vi "test_Basic Deployment.vi"(8 "error in (no error)":errorcluster, 11 "TestCase in":refnum<class "Telemetry System Tests.lvclass">) -> (0 "error out":errorcluster, 3 "TestCase out":refnum<class "Telemetry System Tests.lvclass">)   [LabVIEW 2019, in "Telemetry System Tests.lvclass"]
uses:
  Telemetry System Tests.lvclass
  C:/Users/nitest/Desktop/NI VS Custom Device Testing Tools/VeriStandTestCase/VeriStandTestCase.lvclass
  NI VS Custom Device Testing Tools/VeriStandTestUtilities/TargetPlatform.ctl
  NI VS Custom Device Testing Tools/VeriStandTestUtilities/SystemDefinitionInformation.ctl
  NI VS Custom Device Testing Tools/VeriStandTestUtilities/TargetInformation.ctl
  NI VS Custom Device Testing Tools/VeriStandTestUtilities/ChassisInformation.ctl
  <vilib>/addons/_JKI Toolkits/VI Tester/TestCase.llb/TestCase.lvclass
  TLCD Test/TLCD Test.lvclass
  C:/Program Files (x86)/National Instruments/LabVIEW 2019/vi.lib/addons/_JKI Toolkits/VI Tester/TestCase.llb/TestCase.lvclass
  NI VS Custom Device Testing Tools/VeriStandTestUtilities/VeriStandTestUtilities.lvlib
panel:
  out "System Definition Information":T1
  out "Active Configuration":T4
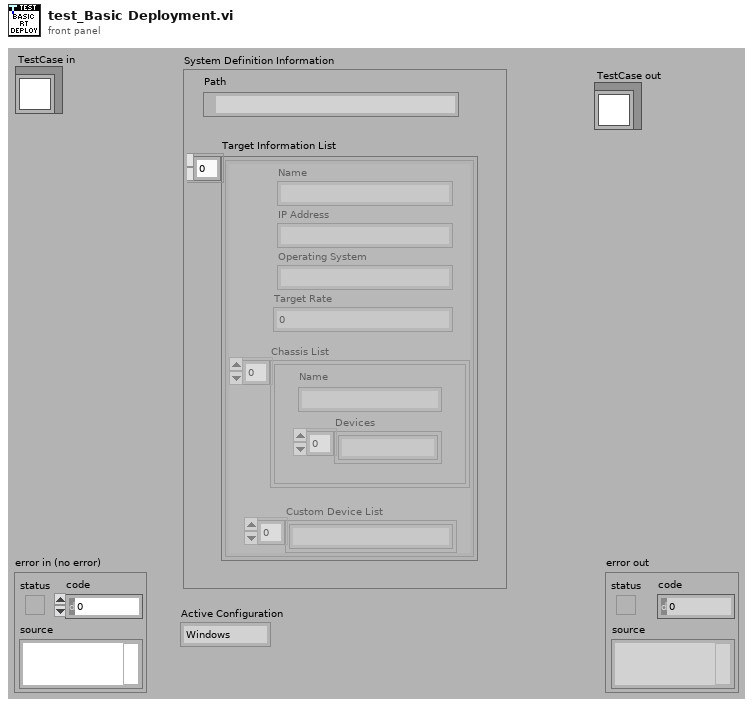
[diagram p1: front panel]
types:
  T1 = typedef "VeriStandTestUtilities.lvlib/SystemDefinitionInformation.ctl" = cluster{"Path":path, "Target Information List":T2[]}
  T2 = typedef "VeriStandTestUtilities.lvlib/TargetInformation.ctl" = cluster{"Name":string, "IP Address":string, "Operating System":string, "Target Rate":dbl, "Chassis List":T3[], "Custom Device List":string[]}
  T3 = typedef "VeriStandTestUtilities.lvlib/ChassisInformation.ctl" = cluster{"Name":string, "Devices":string[]}
  T4 = typedef "VeriStandTestUtilities.lvlib/TargetPlatform.ctl" = enum16{"Windows", "Linux64CRIO", "Linux64PXI", "LinuxARM", "PharLap"}
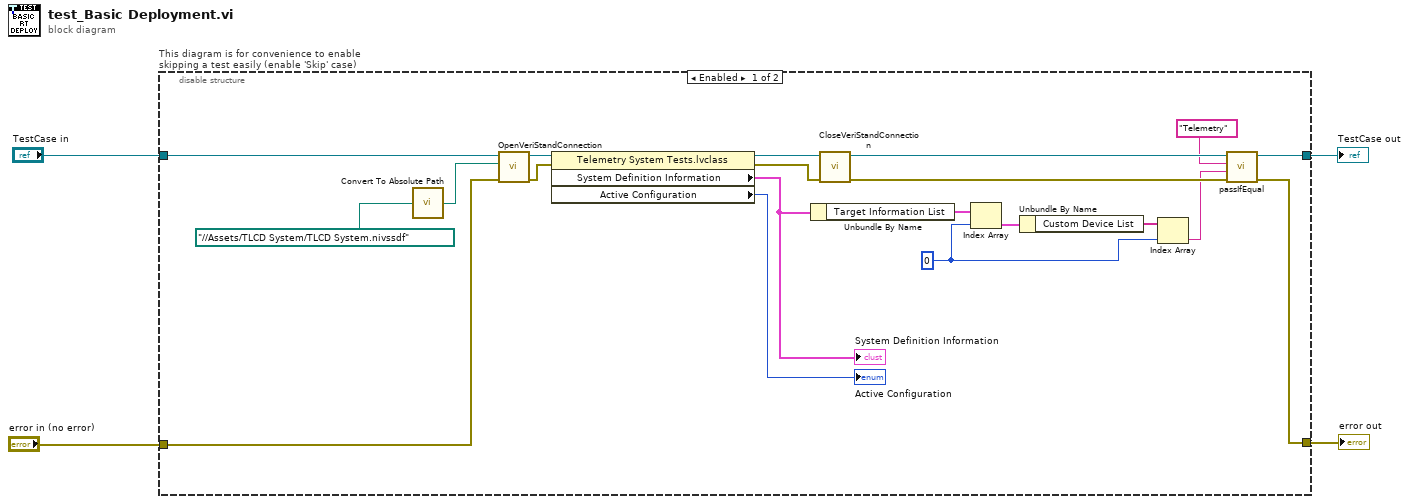
[diagram p0: block diagram]
diagram:
  n1 = disable-structure "This diagram is for convenience to enable skipping a test easily (enable 'Skip' case)" shown="Enabled" {
    disable-tunnel: "TestCase in" -> [w22 w28]
    disable-tunnel: [w6 w26] -> w1
    disable-tunnel: [w5 w27] -> w3
    disable-tunnel: "error in (no error)" -> [w23 w25]
    frame Enabled {
      w11 = 0 ("index")
      n2 = call "Convert To Absolute Path.vi"("System Definition File Path"=path "../../Assets/TLCD System/TLCD System.nivssdf" ("relative base path")) -> ("Absolute path"=w21:path)
      n3 = call-dynamic "OpenVeriStandConnection.vi"("error in (no error)"=w23, "System Definition File"=w21, "VeriStand Test Case in"=w22) -> ("error out"=w17:errorcluster, "VeriStand Test Case out"=w20:refnum<class "Telemetry System Tests.lvclass">)  [unwired: 6 in, 1 out]
      n4 = property class="Telemetry System Tests.lvclass"(reference=w20, error in=w17) -> (reference out=w19:refnum<class "Telemetry System Tests.lvclass">, error out=w15:errorcluster, "System Definition Information"=w16:T1, "Active Configuration"=→"Active Configuration":T4)
      "System Definition Information" <- w16
      n5 = Unbundle By Name(w16) -> ("Target Information List"=w14:T2[])
      n6 = call-dynamic "CloseVeriStandConnection.vi"("error in (no error)"=w15, "VeriStand Test Case in"=w19) -> ("error out"=w9:errorcluster, "VeriStand Test Case out"=w10:refnum<class "Telemetry System Tests.lvclass">)  [unwired: 8 in]
      n7 = Index Array(array=w14, index=w11) -> (element=w13:T2)
      n8 = Unbundle By Name(w13) -> ("Custom Device List"=w12:string[])
      n9 = Index Array(array=w12, index=w11) -> (element=w8:string)
      n10 = call-dynamic "passIfEqual.vi"("error in (no error)"=w9, "y"=w8, "x"="Telemetry" ("element"), "TestCase in"=w10) -> ("error out"=w5:errorcluster, "TestCase out"=w6:refnum<class "Telemetry System Tests.lvclass">)  [unwired: 6 in]
    }
    frame Disabled {
      # "skip test result while test is under development"
      n11 = call <vilib>:"skip.vi"("error in (no error)"=w25, "TestCase in"=w28) -> ("error out"=w27:errorcluster, "TestCase out"=w26:refnum<class "Telemetry System Tests.lvclass">)  [unwired: 8 in]
    }
  }
  "error out" <- w3
  "TestCase out" <- w1
